vi "WriteNetworkSettings.vi"(8 "error in (no error)":errorcluster, 9 "hostname":string, 10 "path":path, 11 "network settings":T1[](array[typedef]) {"IP Address Request Mode" items=["Static"=1, "DHCP/Link Local"=2, "Link-Local Only"=4, "DHCP Only"=8]; "Adapter Mode" items=["Disabled"=1, "TCP/IP Ethernet"=2, "Deterministic"=4, "EtherCAT"=8, "TCP/IP WLAN Connect"=32, "TCP/IP WLAN Create"=64]}) -> (0 "error out":errorcluster)   [LabVIEW 2017, in "USBDrive.lvlib"]
uses:
  <vilib>/addons/InsightCM/Devices/Shared/Common/USBDrive/USBDrive.lvlib
  <vilib>/addons/SystemInfoProcess/controls/NetworkAdapterSettings.ctl
  <vilib>/addons/SystemInfoProcess/SystemInfoProcess.lvlib
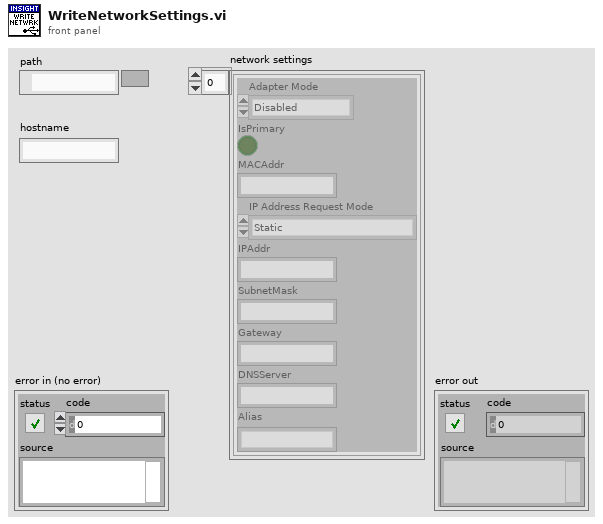
[diagram p1: front panel]
types:
  T1 = typedef "SystemInfoProcess.lvlib/NetworkAdapterSettings.ctl" = cluster{"Adapter Mode":u32, "IsPrimary":bool, "MACAddr":string, "IP Address Request Mode":u32, "IPAddr":string, "SubnetMask":string, "Gateway":string, "DNSServer":string, "Alias":string}
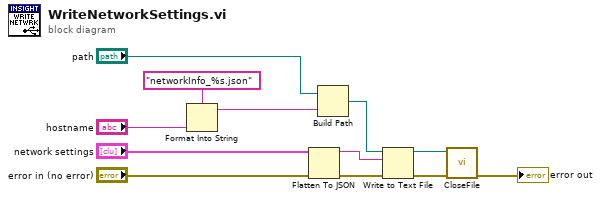
[diagram p0: block diagram]
diagram:
  n1 = Format Into String(format string="networkInfo_%s.json", "hostname") -> (resulting string=w7:string)  [unwired: 2 in, 1 out]
  n2 = Flatten To JSON(anything="network settings", error in (no error)="error in (no error)") -> (JSON string=w10:string, 11:w11:errorcluster)  [unwired: 1 in]
  n3 = Build Path(base path="path", name or relative path=w7) -> (appended path=w12:path)
  n4 = Write to Text File(file (use dialog)=w12, text=w10, error in=w11) -> (refnum out=w3:refnum<file>, error out=w2:errorcluster)  [unwired: 1 in, 1 out]
  n5 = call <vilib>:"CloseFile.vi"("error in (no error)"=w2, "file reference"=w3) -> ("error out"=→"error out":errorcluster)  [unwired: 9 in]
